vi "cmc_selectivechart.vi"() -> ()   [LabVIEW 2010]
panel:
  in  "Boolean":bool
  in  "Delay Time (s)":dbl=1.0
  out "Waveform Chart 2":dbl(graph)
  out "Waveform Chart":dbl(graph)
  in  "stop":bool
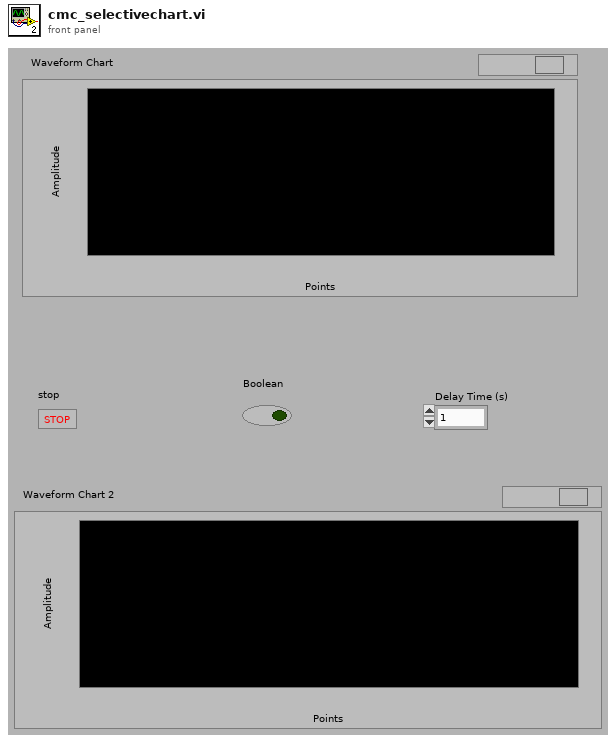
[diagram p1: front panel]
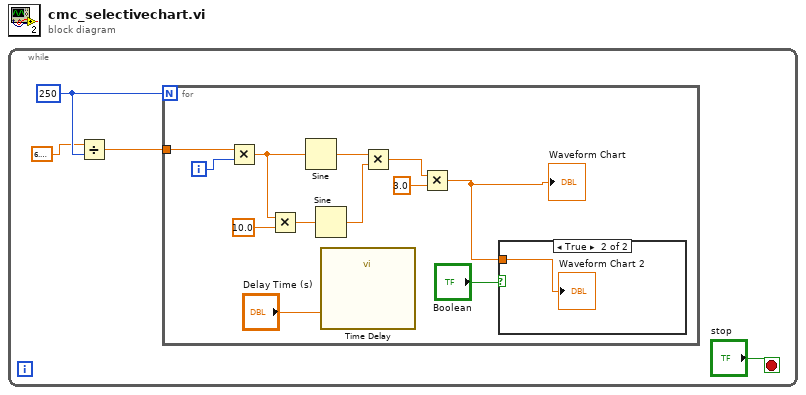
[diagram p0: block diagram]
diagram:
  n1 = while {
    stop <- "stop" stop-if-true
    w2 = 250
    n2 = Divide(x=6.283185307179586, y=w2) -> (x/y=w4:dbl)
    n3 = for {
      N: w2 -> [_]
      tunnel: w4 -> [w16]
      i -> [w15]
      n4 = Multiply(x=w16, y=w15) -> (x*y=w13:dbl)
      n5 = Multiply(x=w13, y=10.0) -> (x*y=w6:dbl)
      n6 = Sine(x=w13) -> (sin(x)=w14:dbl)
      n7 = Sine(x=w6) -> (sin(x)=w5:dbl)
      n8 = call "Time Delay"("Delay Time (s)"="Delay Time (s)") -> ()  [unwired: 10 in, 1 out]
      n9 = Multiply(x=w14, y=w5) -> (x*y=w11:dbl)
      n10 = Multiply(x=w11, y=3.0) -> (x*y=w7:dbl)
      "Waveform Chart" <- w7
      n11 = case shown="True" "Boolean" {
        tunnel: w7 -> [_ w17]
        frame False {
        }
        frame True {
          "Waveform Chart 2" <- w17
        }
      }
    }
  }
